vi "Enum.vi"() -> ()   [LabVIEW 2021]
panel:
  in  "stop":bool
  out "Numeric":i32
  in  "Enum":enum16{"ADD", "Mul", "Division", "Substraction"}(ring)
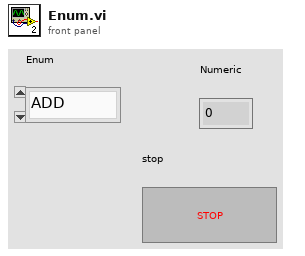
[diagram p1: front panel]
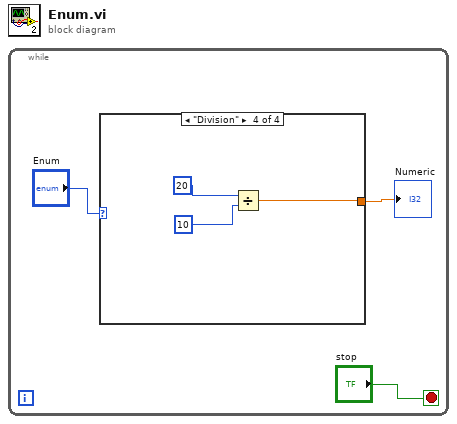
[diagram p0: block diagram]
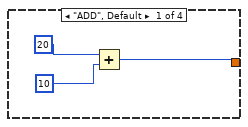
[diagram p2: hidden frame]
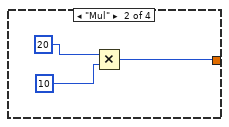
[diagram p3: hidden frame]
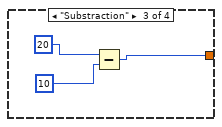
[diagram p4: hidden frame]
diagram:
  n1 = while {
    stop <- "stop" stop-if-true
    n2 = case shown="\"Division\"" "Enum" {
      tunnel: [w4 w7 w10 w13] -> w2
      frame "ADD", Default {
        n3 = Add(x=20, y=10) -> (x+y=w4:i32)
      }
      frame "Mul" {
        n4 = Multiply(x=20, y=10) -> (x*y=w7:i32)
      }
      frame "Substraction" {
        n5 = Subtract(x=20, y=10) -> (x-y=w10:i32)
      }
      frame "Division" {
        n6 = Divide(x=20, y=10) -> (x/y=w13:dbl)
      }
    }
    "Numeric" <- w2
  }
